vi "Write Driver Class.vi"(8 "error in":errorcluster, 10 "Plugin.lvlib:Plugin_Driver.lvclass":refnum<class "Plugin_Driver.lvclass">, 11 "Plugin_Controller in":refnum<class "Plugin_Controller.lvclass">) -> (0 "error out":errorcluster, 3 "Plugin_Controller out":refnum<class "Plugin_Controller.lvclass">)   [LabVIEW 2020, in "Plugin.lvlib" / "Plugin_Controller.lvclass"]
doc: "Write Driver class"
uses:
  Plugin_Controller.lvclass
  Plugin_Driver/Plugin_Driver.lvclass
  Plugin_Controller.lvclass/Plugin_Controller.ctl
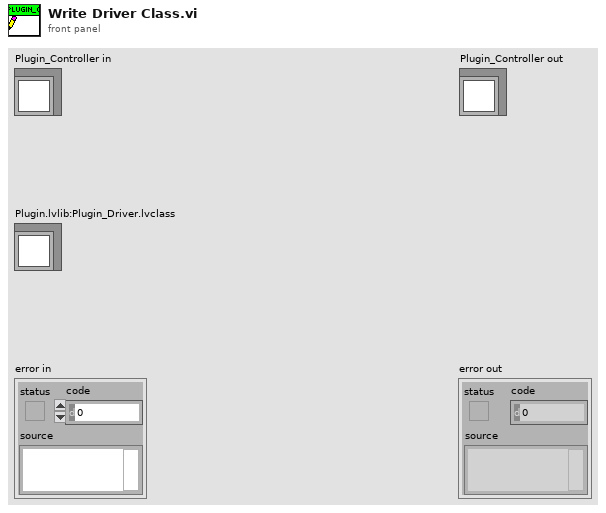
[diagram p1: front panel]
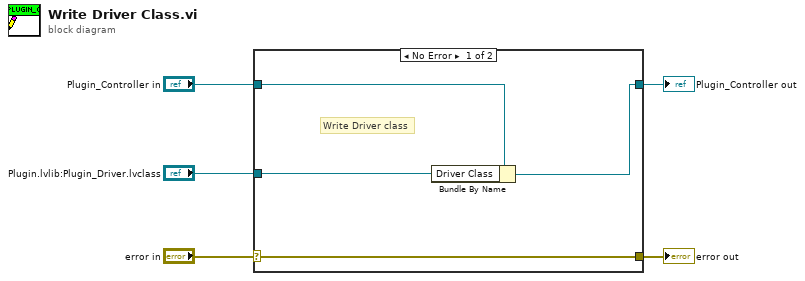
[diagram p0: block diagram]
diagram:
  n1 = case shown="No Error" "error in" {
    selector: "error in" -> [w9 w10]
    tunnel: [w9 w10] -> w4
    tunnel: [w8 w11] -> w2
    tunnel: "Plugin_Controller in" -> [w6 w11]
    tunnel: "Plugin.lvlib:Plugin_Driver.lvclass" -> [w7 _]
    frame No Error {
      # "Write Driver class"
      n2 = Bundle By Name(cluster=w6, "Driver Class"=w7) -> (w8:refnum<class "Plugin_Controller.lvclass">)
    }
    frame Error {
    }
  }
  "error out" <- w4
  "Plugin_Controller out" <- w2
